vi "CANTest2.vi"() -> ()   [LabVIEW 2009]
uses:
  <vilib>/Platform/TimedLoop/XDataNode/XDataNode.xnode
  <vilib>/Platform/TimedLoop/XDataNode/loadlvalarms.vi
  <vilib>/Platform/TimedLoop/XDataNode/timing_clust.ctl
  <vilib>/Platform/TimedLoop/XDataNode/nitl_modes.ctl
  <vilib>/Platform/TimedLoop/XDataNode/wakeup.ctl
  <vilib>/Platform/TimedLoop/XDataNode/XDNodeRunTimeDep.lvlib
  CAN.lvlib
  Serial.lvlib
panel:
  out "read data":u8[](array[numeric]) format="%.0x"
  in  "data":u8[](array[numeric]) format="%.0x"
  in  "messageID":u32 format="%.0x"
  out "error out":errorcluster
  in  "OK Button":bool
  in  "stop 2":bool
  in  "stop":bool
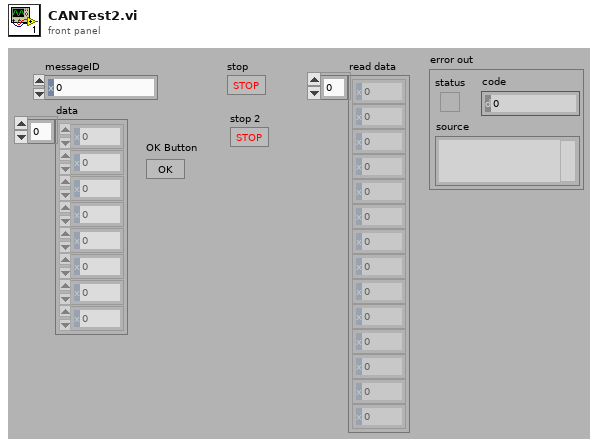
[diagram p1: front panel]
types:
  T1 = typedef "Semaphore RefNum" = refnum<k1>
  T2 = typedef "XDNodeRunTimeDep.lvlib/timing_clust.ctl" = cluster{"Expected End [f-1]":u64, "Actual End [f-1]":u64, "Finished Late? [f-1]":bool, "Expected End [i-1]":u64, "Actual End [i-1]":u64, "Finished Late? [i-1]":bool, "Expected Start [i]":u64, "Actual Start [i]":u64, "Expected Start [f]":u64, "Actual Start [f]":u64, "Source Name":string, "Structure Name":string, "Period":i64, "Deadline":i64, "Offset":i64, "Start":i64, "Priority":i32, "Timeout":i32, "Mode":T3, "Wakeup Reason":T4, "Error":errorcluster, "Source Type":string, "Secondary Source Type":string, "Global End Time":u64, "Global Start Time":u64, "Frame Duration":u64, "Iteration Duration":u64, "Assigned CPU":i32, "I/O Scan Engine Mode":u32}
  T3 = typedef "XDNodeRunTimeDep.lvlib/nitl_modes.ctl" = enum32{"No Change", "Process missed periods, maintain original phase", "Discard missed periods, maintain original phase", "Process missed periods, ignore original phase", "Discard missed periods, ignore original phase"}
  T4 = typedef "XDNodeRunTimeDep.lvlib/wakeup.ctl" = enum32{"Normal", "Aborted", "Asynchronous wakeup", "Timing source error", "Timed loop error", "Timeout"}
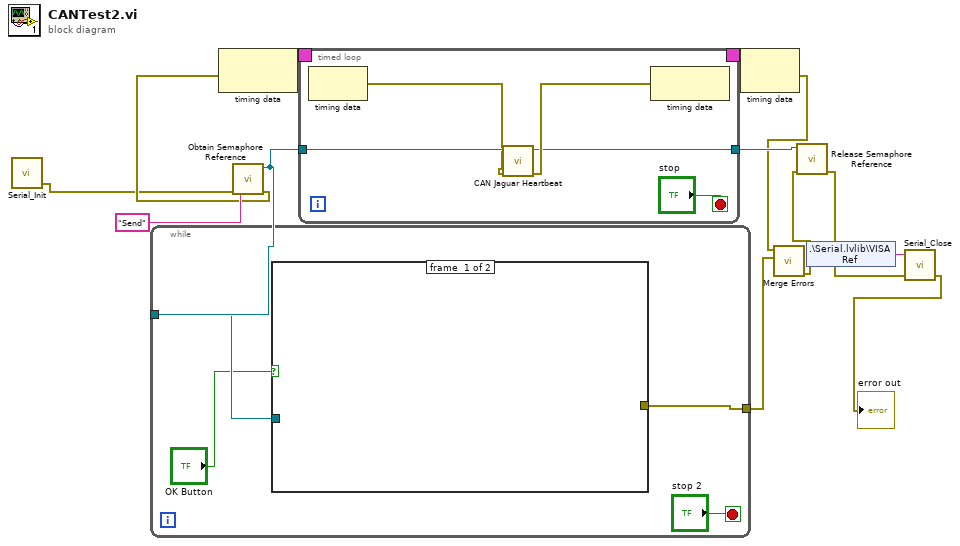
[diagram p0: block diagram]
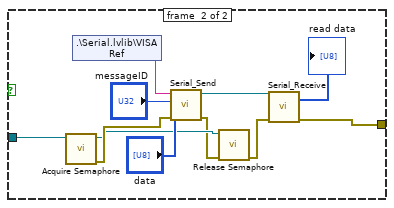
[diagram p2: hidden frame]
diagram:
  n1 = call "Serial_Init.vi"() -> ("error out"=w8:errorcluster)  [unwired: 4 in, 1 out]
  n2 = call <vilib>:"Obtain Semaphore Reference.vi"("error in (no error)"=w8, "name (unnamed)"="Send") -> ("error out"=w10:errorcluster, "semaphore"=w7:T1)  [unwired: 3 in, 1 out]
  n3 = while {
    tunnel: w7 -> [w16]
    tunnel: [w15] -> w6
    stop <- "stop 2" stop-if-true
    n4 = case shown="False" "OK Button" {
      tunnel: w16 -> [_ w19]
      tunnel: [_ w18] -> w15
      frame #0 {
      }
      frame #1 {
        n5 = call <vilib>:"Acquire Semaphore.vi"("semaphore"=w19) -> ("error out"=w25:errorcluster, "semaphore out"=w24:T1)  [unwired: 4 in, 1 out]
        n6 = shared-variable ".\\Serial.lvlib\\VISA Ref"() -> (w28:string)  [unwired: 1 in, 1 out]
        n7 = call "Serial_Send.vi"("error in"=w25, "data"="data", "messageID"="messageID", "VISA resource name"=w28) -> ("error out"=w23:errorcluster, "VISA resource name out"=w21:refnum<visa-resource-name>)  [unwired: 6 in]
        n8 = call <vilib>:"Release Semaphore.vi"("error in (no error)"=w23, "semaphore"=w24) -> ("error out"=w22:errorcluster)  [unwired: 4 in, 1 out]
        n9 = call "Serial_Receive.vi"("error in (no error)"=w22, "VISA resource name"=w21) -> ("error out"=w18:errorcluster, "read data"=→"read data":u8[])  [unwired: 5 in, 3 out]
      }
    }
  }
  n10 = node-c288(w10) -> (w13:T2)
  n11 = timed-loop {
    timing: w13 -> [_]
    timing-out: [_] -> w12
    tunnel: w7 -> [w33]
    tunnel: [w30] -> w9
    stop <- "stop" stop-if-true
    n12 = node-c288() -> (w32:errorcluster)  [unwired: 1 in]
    n13 = call "CAN Jaguar Heartbeat.vi"("error in (no error)"=w32, "semaphore"=w33) -> ("error out"=w31:errorcluster, "semaphore out"=w30:T1)  [unwired: 8 in]
    n14 = node-c288(w31) -> ()  [unwired: 1 out]
  }
  n15 = node-c288(w12) -> (w5:errorcluster)
  n16 = call <vilib>:"Merge Errors.vi"("error in 2 (no error)"=w6, "error in 1 (no error)"=w5) -> ("error out"=w4:errorcluster)  [unwired: 5 in]
  n17 = call <vilib>:"Release Semaphore Reference.vi"("error in (no error)"=w4, "semaphore"=w9) -> ("error out"=w3:errorcluster)  [unwired: 8 in, 1 out]
  n18 = shared-variable ".\\Serial.lvlib\\VISA Ref"() -> (w1:string)  [unwired: 1 in, 1 out]
  n19 = call "Serial_Close.vi"("error in (no error)"=w3, "VISA resource name"=w1) -> ("error out"=→"error out":errorcluster)  [unwired: 3 in]
